vi "Config Process.vi"(8 "error in (no error)":errorcluster, 11 "View Model":T1) -> (0 "error out":errorcluster)   [LabVIEW 2017]
doc: "This process provide operations with configuration database"
uses:
  View Model/Controls/View Model.ctl
  Controls/Config Model.ctl
  Controls/Config Data.ctl
  Error Handler/Controls/Error Model.ctl
  Error Handler/Controls/Error Data.ctl
  Error Handler/Controls/Error Type.ctl
  View Model/Controls/Shared Model.ctl
  Elevator Controller/Controls/Elevator Model.ctl
  Elevator Controller/Controls/Elevator Location.ctl
  Elevator Controller/Controls/Elevator CMD Data.ctl
  Elevator Controller/Controls/Elevator Commands.ctl
  Elevator Controller/Controls/Elevator Overhead.ctl
  Elevator Controller/Controls/Elevator States.ctl
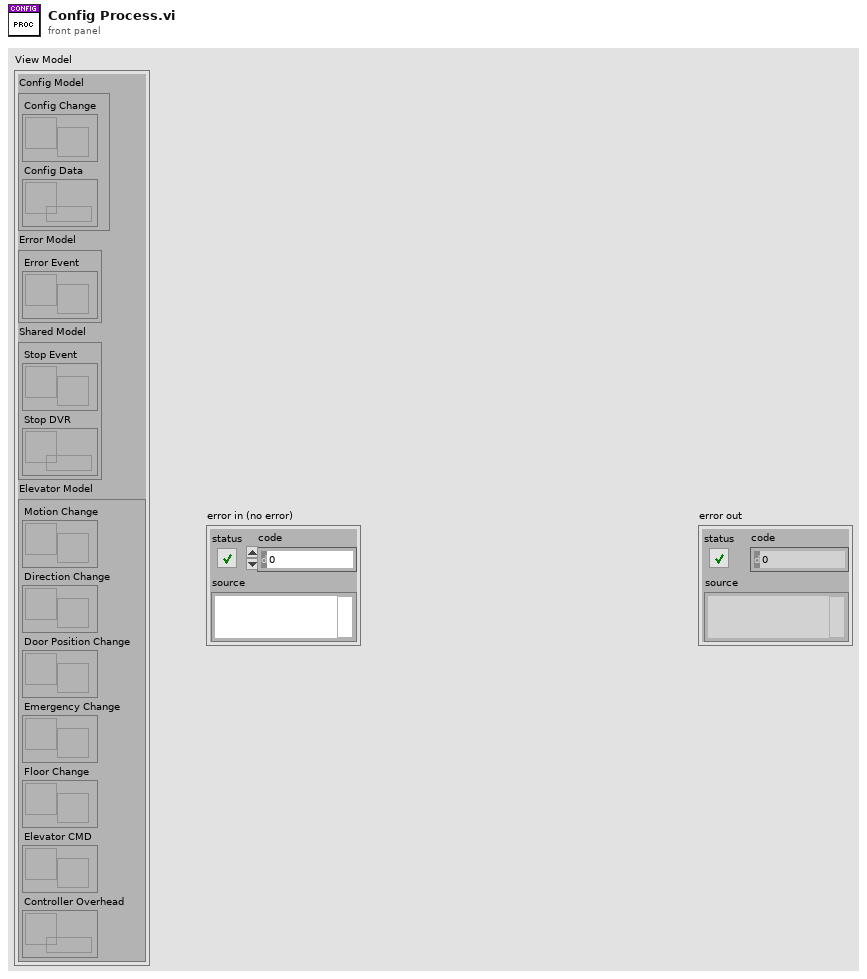
[diagram p1: front panel]
types:
  T1 = typedef "View Model.ctl" = cluster{"Config Model":T2, "Error Model":T3, "Shared Model":T4, "Elevator Model":T5}
  T2 = typedef "Config Model.ctl" = cluster{"Config Change":refnum<user-event>, "Config Data":refnum<data-value>}
  T3 = typedef "Error Model.ctl" = cluster{"Error Event":refnum<user-event>}
  T4 = typedef "Shared Model.ctl" = cluster{"Stop Event":refnum<user-event>, "Stop DVR":refnum<data-value>}
  T5 = typedef "Elevator Model.ctl" = cluster{"Motion Change":refnum<user-event>, "Direction Change":refnum<user-event>, "Door Position Change":refnum<user-event>, "Emergency Change":refnum<user-event>, "Floor Change":refnum<user-event>, "Elevator CMD":refnum<user-event>, "Controller Overhead":refnum<data-value>}
  T6 = typedef "Config Data.ctl" = cluster{"Door Open":dbl, "Door Close":dbl, "Travel Time":dbl, "Inactivity Time":dbl}
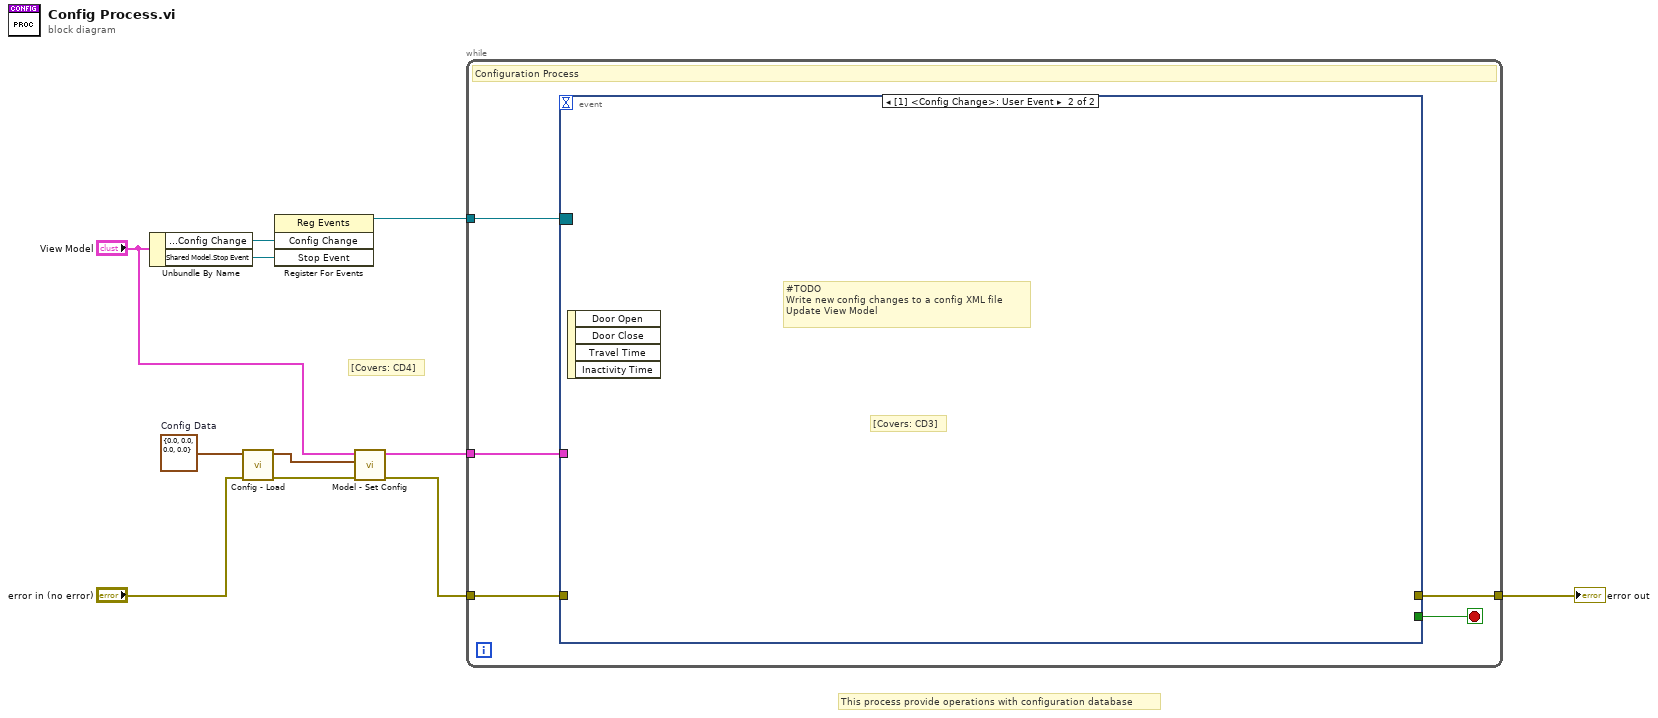
[diagram p0: block diagram]
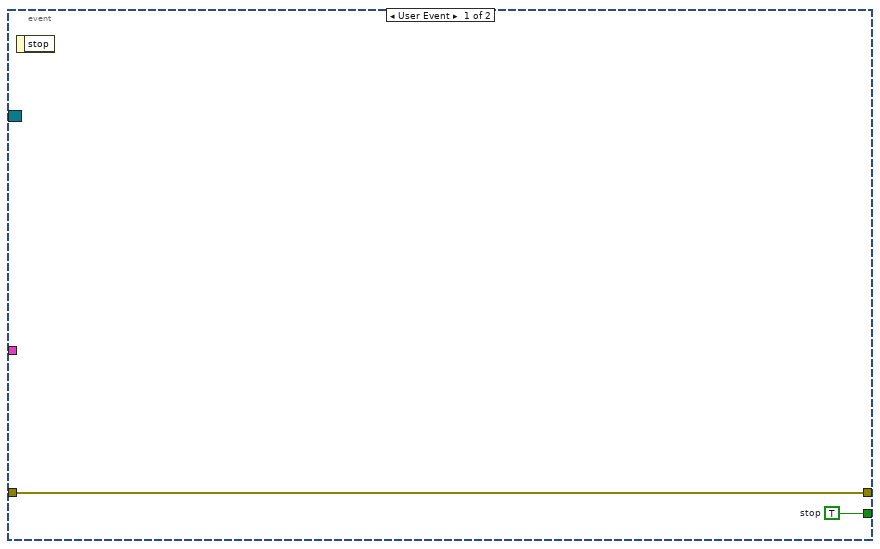
[diagram p2: hidden frame]
diagram:
  w7 = T6 {"Door Open"=0.0, "Door Close"=0.0, "Travel Time"=0.0, "Inactivity Time"=0.0}  # Config Data
  # "This process provide operations with configuration database"
  # "[Covers: CD4]"
  n1 = Unbundle By Name("View Model") -> ("Config Model.Config Change"=w11:refnum<user-event>, "Shared Model.Stop Event"=w10:refnum<user-event>)
  n2 = call "Config - Load.vi"("error in (no error)"="error in (no error)", "Config Data"=w7) -> ("error out"=w3:errorcluster, "Config Data"=w5:T6)  [unwired: 8 in]
  n3 = register-events(w11, w10) -> (reference out=w9:refnum<event-registration>)  [unwired: 2 in, 1 out]
  n4 = call "Model - Set Config.vi"("error in (no error)"=w3, "Configuration"=w5, "View Model"="View Model") -> ("error out"=w2:errorcluster, "View Model"=w1:T1)  [unwired: 7 in]
  n5 = while {
    tunnel: w9 -> [w16]
    tunnel: w2 -> [w15]
    tunnel: [w14] -> w8
    tunnel: w1 -> [w12]
    stop <- w13 stop-if-true
    # "Configuration Process"
    n6 = event shown="[1] <Config Change>: User Event" {
      selector: w16 -> [_ _]
      dyn-events: _ -> [_ _]
      timeout: _ -> [_ _]
      tunnel: w15 -> [w17 _]
      tunnel: [w17 _] -> w14
      tunnel: [w18 _] -> w13
      tunnel: w12 -> [_ _]
      event User Event {
        w18 = TRUE  # stop
        n7 = event-data() -> ()  [unwired: 1 in, 1 out]
      }
      event User Event {
        # "[Covers: CD3]"
        # "#TODO\nWrite new config changes to a config XML file\nUpdate View Model"
        n8 = event-data() -> ()  [unwired: 1 in, 4 out]
      }
    }
  }
  "error out" <- w8
